vi "FPGAcode3.vi"() -> ()   [LabVIEW 2015]
uses:
  <vilib>/Platform/TimedLoop/XDataNode/wakeup.ctl
  <vilib>/Platform/TimedLoop/XDataNode/XDNodeRunTimeDep.lvlib
  <vilib>/Platform/TimedLoop/XDataNode/nitl_modes.ctl
  <vilib>/Platform/TimedLoop/XDataNode/timing_clust.ctl
  <vilib>/Platform/TimedLoop/XDataNode/XDataNode.xnode
  <vilib>/eio/EIONode/EIONode.xnode
  <vilib>/rvi/eio/common/nirviEmuTemplateMethod_errors.vi
  Detector_Cluster.ctl
  Limits_In.ctl
panel:
  out "DCS 1":bool
  in  "Limits":T1
  in  "Filter Thresholds":T2
  out "Detector 3 Max Correlations":T2
  out "Detector 3 Correlations":T2
  out "Detector 1 Correlations":T2
  in  "Calibrate":bool
  out "IO Module\\AI 1":i16
  out "IO Module\\AI 0":i16
  out "Armed":bool
  out "Plates":bool
  in  "One Shot":bool
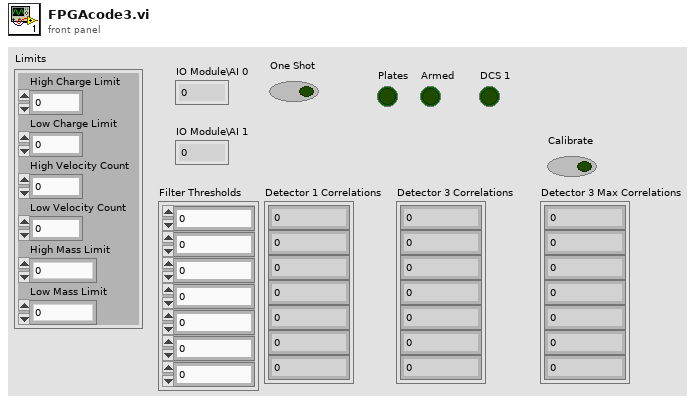
[diagram p1: front panel]
types:
  T1 = typedef "Limits_In.ctl" = cluster{"High Charge Limit":i16, "Low Charge Limit":i16, "High Velocity Count":i32, "Low Velocity Count":i32, "High Mass Limit":i64, "Low Mass Limit":i64}
  T2 = typedef "Detector_Cluster.ctl" = cluster{"1":i32, "2":i32, "3":i32, "4":i32, "5":i32, "6":i32, "7":i32}
  T3 = typedef "XDNodeRunTimeDep.lvlib/timing_clust.ctl" = cluster{"Expected End [f-1]":u64, "Actual End [f-1]":u64, "Finished Late? [f-1]":bool, "Expected End [i-1]":u64, "Actual End [i-1]":u64, "Finished Late? [i-1]":bool, "Expected Start [i]":u64, "Actual Start [i]":u64, "Expected Start [f]":u64, "Actual Start [f]":u64, "Source Name":string, "Structure Name":string, "Period":i64, "Deadline":i64, "Offset":i64, "Start":i64, "Priority":i32, "Timeout":i32, "Mode":T4, "Wakeup Reason":T5, "Error":errorcluster, "Source Type":string, "Secondary Source Type":string, "Global End Time":u64, "Global Start Time":u64, "Frame Duration":u64, "Iteration Duration":u64, "Assigned CPU":i32, "I/O Scan Engine Mode":u32}
  T4 = typedef "XDNodeRunTimeDep.lvlib/nitl_modes.ctl" = enum32{"No Change", "Process missed periods, maintain original phase", "Discard missed periods, maintain original phase", "Process missed periods, ignore original phase", "Discard missed periods, ignore original phase"}
  T5 = typedef "XDNodeRunTimeDep.lvlib/wakeup.ctl" = enum32{"Normal", "Aborted", "Asynchronous wakeup", "Timing source error", "Timed loop error", "Timeout"}
  T6 = cluster{"High Charge Limit":i16, "Low Charge Limit":i16, "Time Out Limit":u32, "High Velocity Count":i32, "Low Velocity Count":i32, "Sampling Rate":fxp<+,30,25>, "High Mass Limit":i64, "Low Mass Limit":i64}
  T7 = cluster{"[0]":i32, "[1]":i32, "[2]":i32, "[3]":i32, "[4]":i32, "[5]":i32, "[6]":i32}
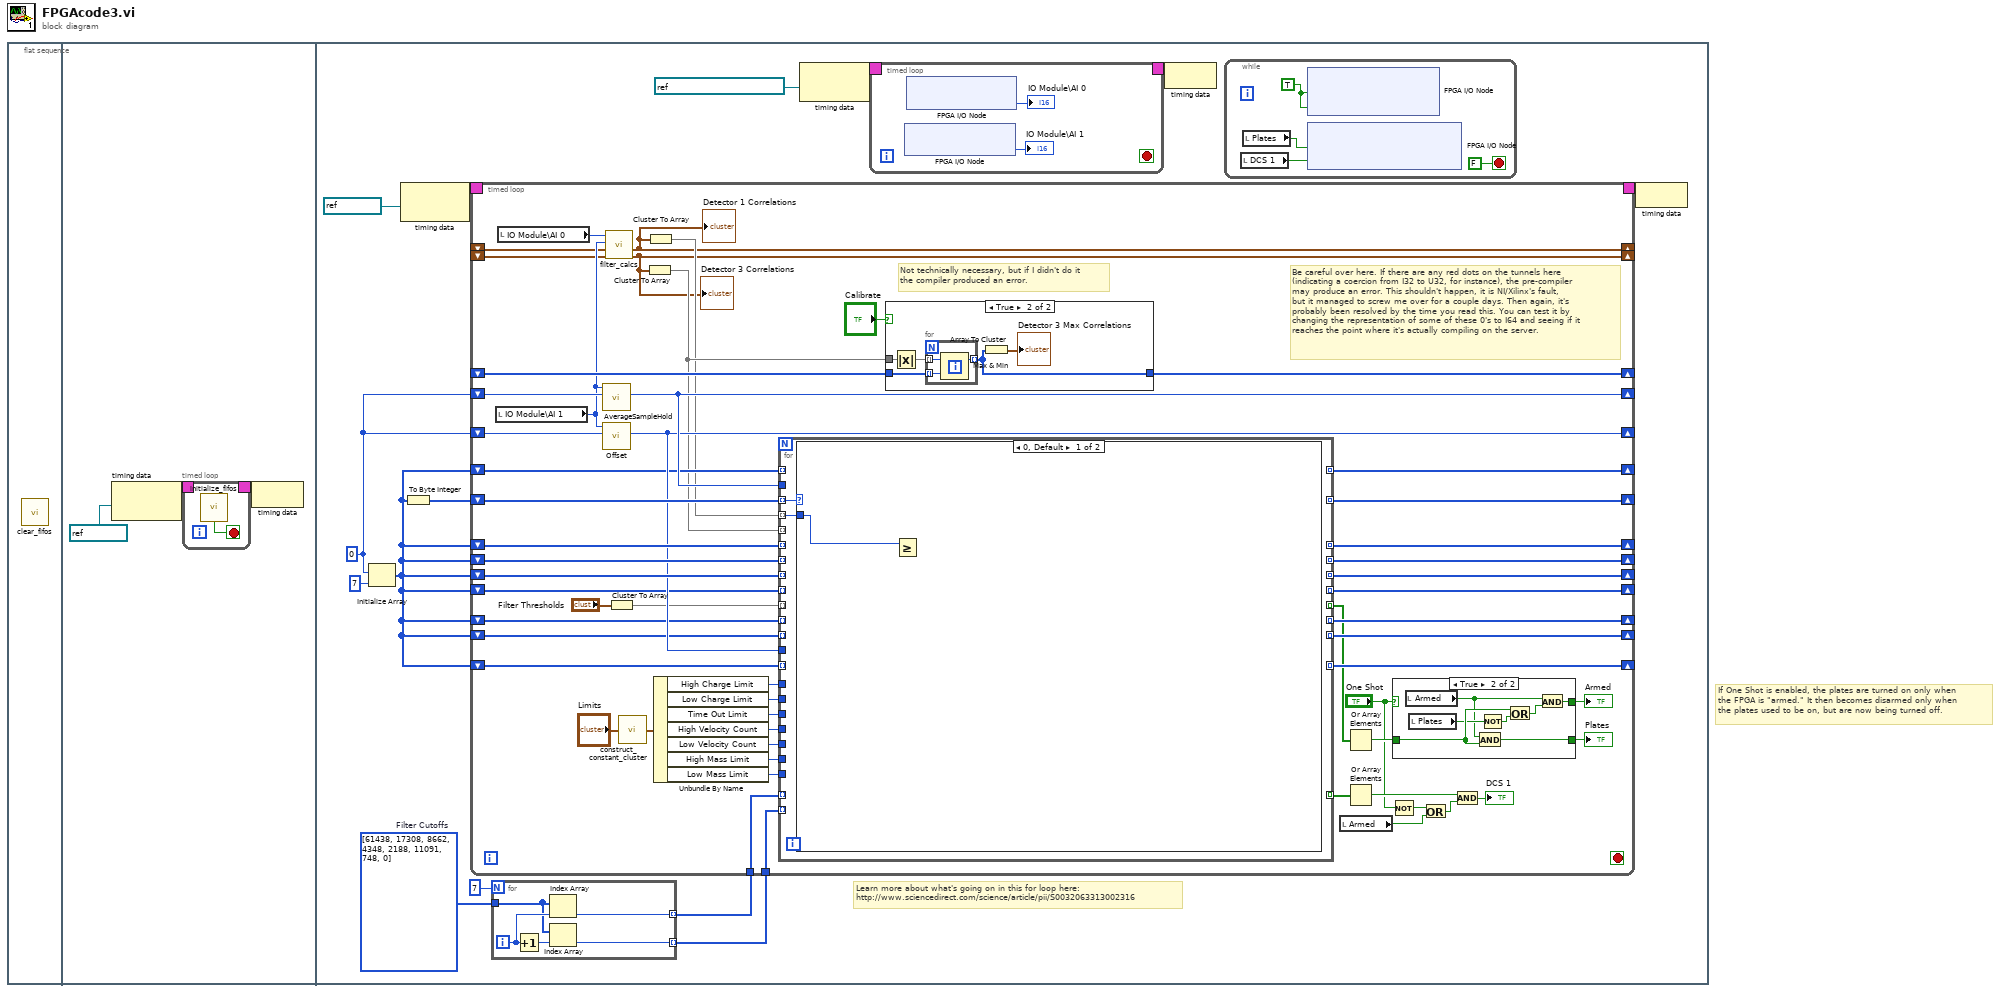
[diagram p0: block diagram]
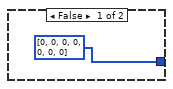
[diagram p2: hidden frame]
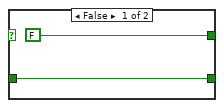
[diagram p3: hidden frame]
diagram:
  # "If One Shot is enabled, the plates are turned on only when\nthe FPGA is \"armed.\" It then becomes disarmed only when\nthe plates used to be on, but are now being turned off."
  n1 = flat-sequence {
    frame #0 {
      n2 = call "clear_fifos.vi"() -> ()  [unwired: 1 in]
    }
    frame #1 {
      n3 = node-c288(refnum<k21> "50MHz" ("Source Name")) -> (w3:T3)
      n4 = timed-loop {
        timing: w3 -> [_]
        timing-out: [_] -> w2
        stop <- w4 stop-if-true
        n5 = call "initialize_fifos.vi"() -> ("Output State"=w4:bool)
      }
      n6 = node-c288(w2) -> ()
    }
    frame #2 {
      w11 = i32[] [61438, 17308, 8662, 4348, 2188, 11091, 748, 0]  # Filter Cutoffs
      w13 = 0 ("Output New Average")
      # "Learn more about what's going on in this for loop here:\nhttp://www.sciencedirect.com/science/article/pii/S0032063313002316"
      n7 = Initialize Array(w13, 7 ("dimension size")) -> (w14:i32[])
      n8 = node-c288(refnum<k21> "50MHz" ("Source Name")) -> (w24:T3)
      n9 = To Byte Integer(number=w14) -> (8bit integer=w12:i8[])
      n10 = for {
        N: 7 -> [_]
        tunnel: w11 -> [w27]
        tunnel: [w26] -> w17 mode=indexing
        tunnel: [w25] -> w16 mode=indexing
        i -> [w29]
        n11 = Increment(x=w29) -> (x+1=w28:i32)
        n12 = Index Array(array=w27, index=w29) -> (element=w26:i32)
        n13 = Index Array(array=w27, index=w28) -> (element=w25:i32)
      }
      n14 = timed-loop {
        timing: w24 -> [_]
        timing-out: [_] -> w23
        shift-right: [w97] -> _
        shift-left: w13 -> [w98]
        shift-right: [w95] -> _
        shift-left: w12 -> [w96]
        shift-right: [w85] -> _
        shift-left: w14 -> [w94]
        shift-right: [w84] -> _
        shift-left: w14 -> [w93]
        shift-right: [w83] -> _
        shift-left: w14 -> [w92]
        shift-right: [w79] -> _
        shift-left: w14 -> [w91]
        shift-right: [w89] -> _
        shift-left: w13 -> [w90]
        shift-right: [w82] -> _
        shift-left: w14 -> [w88]
        shift-right: [w81] -> _
        shift-left: w14 -> [w87]
        shift-right: [w80] -> _
        shift-left: w14 -> [w86]
        tunnel: w17 -> [w77]
        tunnel: w16 -> [w76]
        shift-right: [w74] -> _
        shift-left: w14 -> [w75]
        shift-right: [w62] -> _
        shift-left: _ -> [w61]
        shift-right: [w53] -> _
        shift-left: _ -> [w51]
        shift-right: [w52] -> _
        shift-left: _ -> [w50]
        stop <- _ stop-if-true
        # "Be careful over here. If there are any red dots on the tunnels here\n(indicating a coercion from I32 to U32, for instance), the pre-compiler\nmay produce an error. This shouldn't happen, it is NI/Xilinx's fault,\nbut it managed to screw me over for a couple days. Then again, it's\nprobably been resolved by the time you read this. You can test it by\nchanging the representation of some of these 0's to I64 and seeing if it\nreaches the point where it's actually compiling on the server."
        # "Not technically necessary, but if I didn't do it\nthe compiler produced an error."
        n15 = local read "IO Module\\AI 1"() -> (w55:i16)
        n16 = local read "IO Module\\AI 0"() -> (w54:i16)
        n17 = call "AverageSampleHold.vi"("Previous Average"=w98, "Input Value"=w55) -> ("Output New Average"=w97:i32)  [unwired: 9 in]
        n18 = call "Offset.vi"("Previous Average"=w90, "Input Value"=w55) -> ("Output New Average"=w89:i32)  [unwired: 9 in]
        n19 = call "filter_calcs.vi"("Detector 3 Correlations In"=w50, "Detector 1 Correlations In"=w51, "Detector 3"=w55, "Detector 1"=w54) -> ("Detector 3 Correlations Out"=w52:T2, "Detector 1 Correlations Out"=w53:T2)  [unwired: 6 in]
        "Detector 1 Correlations" <- w53
        "Detector 3 Correlations" <- w52
        n20 = Cluster To Array(cluster="Filter Thresholds") -> (array=w49:i32[])
        n21 = call "construct_constant_cluster.vi"("Cluster"="Limits") -> ("Limits"=w59:T6)
        n22 = Cluster To Array(cluster=w52) -> (array=w57:i32[])
        n23 = Cluster To Array(cluster=w53) -> (array=w56:i32[])
        n24 = Unbundle By Name(w59) -> ("High Charge Limit"=w64:i16, "Low Charge Limit"=w65:i16, "Time Out Limit"=w66:u32, "High Velocity Count"=w67:i32, "Low Velocity Count"=w68:i32, "High Mass Limit"=w69:i64, "Low Mass Limit"=w70:i64)
        n25 = for {
          tunnel: w56 -> [w117] mode=indexing
          tunnel: w57 -> [_] mode=indexing
          tunnel: w75 -> [_] mode=indexing
          tunnel: [_] -> w74 mode=indexing
          tunnel: w96 -> [w118] mode=indexing
          tunnel: [_] -> w95 mode=indexing
          tunnel: w94 -> [_] mode=indexing
          tunnel: w93 -> [_] mode=indexing
          tunnel: w92 -> [_] mode=indexing
          tunnel: w91 -> [_] mode=indexing
          tunnel: w88 -> [_] mode=indexing
          tunnel: w49 -> [_] mode=indexing
          tunnel: w87 -> [_] mode=indexing
          tunnel: w86 -> [_] mode=indexing
          tunnel: [_] -> w85 mode=indexing
          tunnel: [_] -> w84 mode=indexing
          tunnel: [_] -> w83 mode=indexing
          tunnel: [_] -> w82 mode=indexing
          tunnel: [_] -> w81 mode=indexing
          tunnel: [_] -> w80 mode=indexing
          tunnel: [_] -> w79 mode=indexing
          tunnel: [_] -> w73 mode=indexing
          tunnel: w97 -> [_]
          tunnel: w89 -> [_]
          tunnel: w77 -> [_] mode=indexing
          tunnel: w76 -> [_] mode=indexing
          tunnel: w70 -> [_]
          tunnel: w69 -> [_]
          tunnel: w68 -> [_]
          tunnel: w67 -> [_]
          tunnel: w66 -> [_]
          tunnel: w65 -> [_]
          tunnel: w64 -> [_]
          tunnel: [_] -> w48 mode=indexing
          n26 = case shown="0, Default" w118 {
            tunnel: w117 -> [w119 _]
            frame 0, Default {
              n27 = Greater Or Equal?(x=w119) -> ()  [unwired: 1 in, 1 out]
            }
            frame 1 {
            }
          }
        }
        n28 = case shown="True" "Calibrate" {
          tunnel: w57 -> [_ w103]
          tunnel: w61 -> [_ w102]
          tunnel: [i16[] [0, 0, 0, 0, 0, 0, 0] w101] -> w62
          frame False {
          }
          frame True {
            n29 = Absolute Value(x=w103) -> (abs(x)=w100:i32[])
            n30 = for {
              tunnel: w102 -> [w107] mode=indexing
              tunnel: [w106] -> w101 mode=indexing
              tunnel: w100 -> [w105] mode=indexing
              n31 = Max & Min(x=w105, y=w107) -> (max(x,y)=w106:i32)  [unwired: 1 out]
            }
            n32 = Array To Cluster(array=w101) -> (cluster=→"Detector 3 Max Correlations":T7)
          }
        }
        n33 = local read "Armed"() -> (w43:bool)
        n34 = Or Array Elements(Boolean array=w73) -> (logical OR=w72:bool)
        n35 = Or Array Elements(Boolean array=w48) -> (logical OR=w47:bool)
        n36 = Not(x="One Shot") -> (.not. x?=w42:bool)
        n37 = case shown="True" "One Shot" {
          tunnel: [w109 w115] -> w78
          tunnel: w72 -> [w109 w112]
          tunnel: [FALSE w116] -> w71
          frame False {
          }
          frame True {
            n38 = local read "Armed"() -> (w110:bool)
            n39 = local read "Plates"() -> (w111:bool)
            n40 = And(x=w110, y=w112) -> (x .and. y?=w115:bool)
            n41 = Not(x=w111) -> (.not. x?=w113:bool)
            n42 = Or(x=w112, y=w113) -> (x .or. y?=w114:bool)
            n43 = And(x=w110, y=w114) -> (x .and. y?=w116:bool)
          }
        }
        "Plates" <- w78
        "Armed" <- w71
        n44 = Or(x=w42, y=w43) -> (x .or. y?=w45:bool)
        n45 = And(x=w47, y=w45) -> (x .and. y?=→"DCS 1":bool)
      }
      n46 = node-c288(refnum<k21> "IO Module\\Data Clock" ("Source Name")) -> (w21:T3)
      n47 = timed-loop {
        timing: w21 -> [_]
        timing-out: [_] -> w20
        stop <- _ stop-if-true
        n48 = xnode "FPGA I/O Node"() -> ("IO Module\\AI 1"=→"IO Module\\AI 1":i16)  [unwired: 1 in, 1 out]
        n49 = xnode "FPGA I/O Node"() -> ("IO Module\\AI 0"=→"IO Module\\AI 0":i16)  [unwired: 1 in, 1 out]
      }
      n50 = node-c288(w20) -> ()
      n51 = while {
        stop <- FALSE stop-if-true
        w40 = TRUE ("IO Module\\PFI Enable")
        n52 = local read "DCS 1"() -> (w38:bool)
        n53 = local read "Plates"() -> (w39:bool)
        n54 = xnode "FPGA I/O Node"("IO Module\\PFI 0 WE"=w40, "IO Module\\PFI 1 WE"=w40) -> ()  [unwired: 2 in, 2 out]
        n55 = xnode "FPGA I/O Node"("IO Module\\PFI 0 Wr Data"=w39, "IO Module\\PFI 1 Wr Data"=w38) -> ()  [unwired: 2 in, 2 out]
      }
      n56 = node-c288(w23) -> ()
    }
  }
